vi "Parse Value.vi"(8 "error in (no error)":errorcluster, 10 "Index In":i32, 11 "JSON String":string) -> (0 "error out":errorcluster, 2 "Index Out":i32, 3 "JSON Value out":variant)   [LabVIEW 2017, in "Advanced Variant Tools.lvlib"]
uses:
  Advanced Variant Tools.lvlib
  Errors.ctl
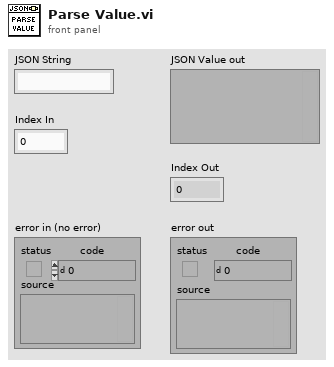
[diagram p1: front panel]
types:
  T1 = typedef "Advanced Variant Tools.lvlib/Errors.ctl" = enum16{"No key", "Key path type", "Array OOB", "Type Mismatch", "Invalid Token", "Invalid Value"}
  T2 = typedef "Advanced Variant Tools.lvlib/Token Type.ctl" = enum16{"NONE", "CURLY_OPEN", "CURLY_CLOSE", "SQUARED_OPEN", "SQUARED_CLOSE", "COLON", "COMMA", "STRING", "NUMBER", "TRUE", "FALSE", "NULL"}
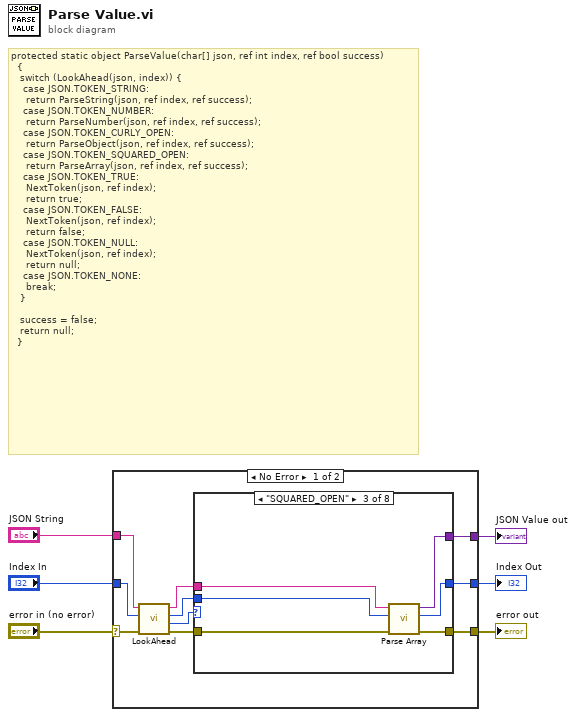
[diagram p0: block diagram]
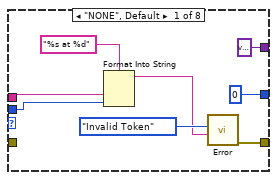
[diagram p2: hidden frame]
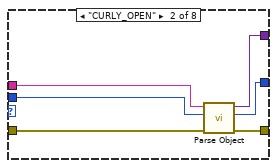
[diagram p3: hidden frame]
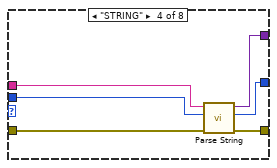
[diagram p4: hidden frame]
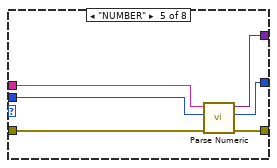
[diagram p5: hidden frame]
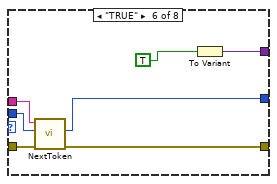
[diagram p6: hidden frame]
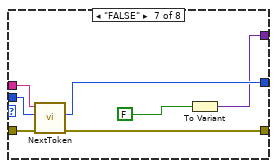
[diagram p7: hidden frame]
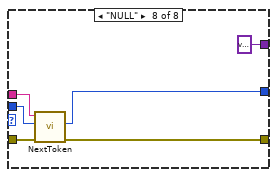
[diagram p8: hidden frame]
diagram:
  # "protected static object ParseValue(char[] json, ref int index, ref bool success)\n\t\t{\n\t\t\tswitch (LookAhead(json, index)) {\n\t\t\t\tcase JSON.TOKEN_STRING:\n\t\t\t\t\treturn ParseString(json, ref index, ref success);\n\t\t\t\tcase JSON.TOKEN_NUMBER:\n\t\t\t\t\treturn ParseNumber(json, ref index, ref success);\n\t\t\t\tcase JSON.TOKEN_CURLY_OPEN:\n\t\t\t\t\treturn ParseObject(json, ref index, ref success);\n\t\t\t\tcase JSON.TOKEN_SQUARED_OPEN:\n\t\t\t\t\treturn ParseArray(json, ref index, ref success);\n\t\t\t\tcase JSON.TOKEN_TRUE:\n\t\t\t\t\tNextToken(json, ref index);\n\t\t\t\t\treturn true;\n\t\t\t\tcase JSON.TOKEN_FALSE:\n\t\t\t\t\tNextToken(json, ref index);\n\t\t\t\t\treturn false;\n\t\t\t\tcase JSON.TOKEN_NULL:\n\t\t\t\t\tNextToken(json, ref index);\n\t\t\t\t\treturn null;\n\t\t\t\tcase JSON.TOKEN_NONE:\n\t\t\t\t\tbreak;\n\t\t\t}\n\n\t\t\tsuccess = false;\n\t\t\treturn null;\n\t\t}"
  n1 = case shown="No Error" "error in (no error)" {
    selector: "error in (no error)" -> [w16 w69]
    tunnel: [w14 w69] -> w5
    tunnel: "JSON String" -> [w10 _]
    tunnel: "Index In" -> [w9 _]
    tunnel: [w8 _] -> w1
    tunnel: [w7 _] -> w2
    frame No Error {
      n2 = call "LookAhead.vi"("error in (no error)"=w16, "Index"=w9, "JSON String"=w10) -> ("error out"=w15:errorcluster, "TOKEN"=w13:T2, "Index Passthrough"=w11:i32, "JSON String Passthrough"=w12:string)  [unwired: 5 in]
      n3 = case shown="\"SQUARED_OPEN\"" w13 {
        tunnel: w15 -> [_ w28 w34 w40 w46 w52 w61 w65]
        tunnel: [w23 w27 w33 w39 w45 w51 w58 w68] -> w14
        tunnel: [variant ("Variant") w25 w31 w37 w43 w49 w56 variant ("Variant")] -> w8
        tunnel: w12 -> [w20 w29 w36 w42 w48 w55 w59 w67]
        tunnel: w11 -> [w19 w30 w35 w41 w47 w54 w60 w66]
        tunnel: [0 ("Index Out") w26 w32 w38 w44 w53 w62 w64] -> w7
        frame "NONE", Default {
          n4 = Format Into String(format string="%s at %d", w20, w19) -> (resulting string=w18:string)  [unwired: 2 in, 1 out]
          n5 = call "Error.vi"("Data"=w18, 9:Errors."Invalid Token") -> ("error out"=w23:errorcluster)  [unwired: 8 in]
        }
        frame "CURLY_OPEN" {
          n6 = call "Parse Object.vi"("error in (no error)"=w28, "Index In"=w30, "JSON String"=w29) -> ("error out"=w27:errorcluster, "Index Out"=w26:i32, "JSON Value out"=w25:variant)  [unwired: 6 in]
        }
        frame "SQUARED_OPEN" {
          n7 = call "Parse Array.vi"("error in (no error)"=w34, "Index In"=w35, "JSON String"=w36) -> ("error out"=w33:errorcluster, "Index Out"=w32:i32, "JSON Value out"=w31:variant)  [unwired: 6 in]
        }
        frame "STRING" {
          n8 = call "Parse String.vi"("error in (no error)"=w40, "Index In"=w41, "JSON String"=w42) -> ("error out"=w39:errorcluster, "Index Out"=w38:i32, "JSON Value out"=w37:variant)  [unwired: 5 in, 1 out]
        }
        frame "NUMBER" {
          n9 = call "Parse Numeric.vi"("error in (no error)"=w46, "Index In"=w47, "JSON String"=w48) -> ("error out"=w45:errorcluster, "Index Out"=w44:i32, "JSON Value out"=w43:variant)  [unwired: 6 in]
        }
        frame "TRUE" {
          n10 = call "NextToken.vi"("error in (no error)"=w52, "Index In"=w54, "JSON String"=w55) -> ("error out"=w51:errorcluster, "Index Out"=w53:i32)  [unwired: 5 in, 2 out]
          n11 = To Variant(anything=TRUE) -> (Variant=w49:variant)
        }
        frame "FALSE" {
          n12 = call "NextToken.vi"("error in (no error)"=w61, "Index In"=w60, "JSON String"=w59) -> ("error out"=w58:errorcluster, "Index Out"=w62:i32)  [unwired: 5 in, 2 out]
          n13 = To Variant(anything=FALSE) -> (Variant=w56:variant)
        }
        frame "NULL" {
          n14 = call "NextToken.vi"("error in (no error)"=w65, "Index In"=w66, "JSON String"=w67) -> ("error out"=w68:errorcluster, "Index Out"=w64:i32)  [unwired: 5 in, 2 out]
        }
      }
    }
    frame Error {
    }
  }
  "error out" <- w5
  "Index Out" <- w2
  "JSON Value out" <- w1
